vi "VIRefToJson.vi"(8 "error (in)":errorcluster, 10 "Destination Directory":path, 11 "vi reference":refnum<vi>) -> (0 "error out":errorcluster, 2 "JSON File Path":path, 3 "JSON":string)   [LabVIEW 2017]
panel:
  out "resulting string":string
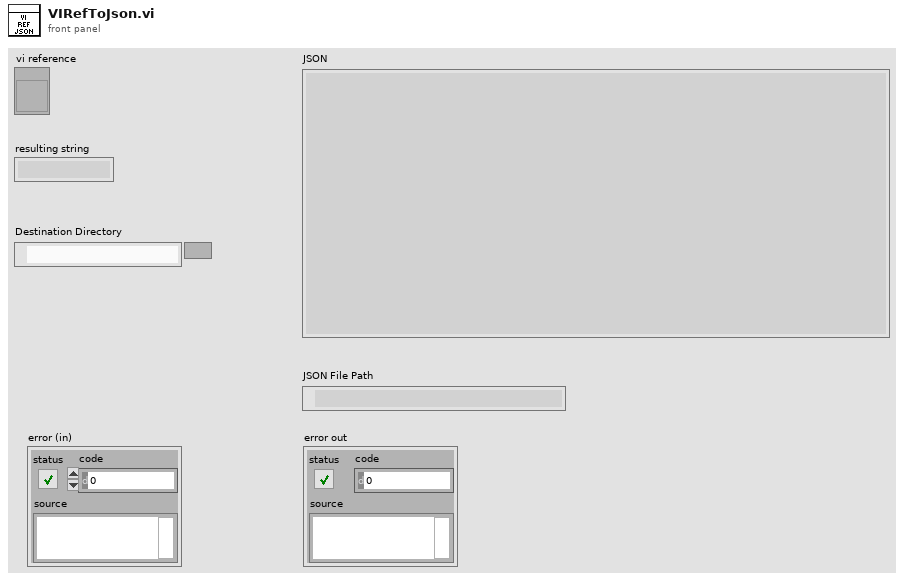
[diagram p1: front panel]
types:
  T1 = enum32{"invalid VI type", "Standard VI", "Control VI", "Global VI", "Polymorphic VI", "Configuration VI", "SubSystem", "Facade VI", "Method VI", "Statechart Diagram VI"}
  T2 = cluster{"VIPath":path, "Menu Name":string, "Selector Name":string}[]
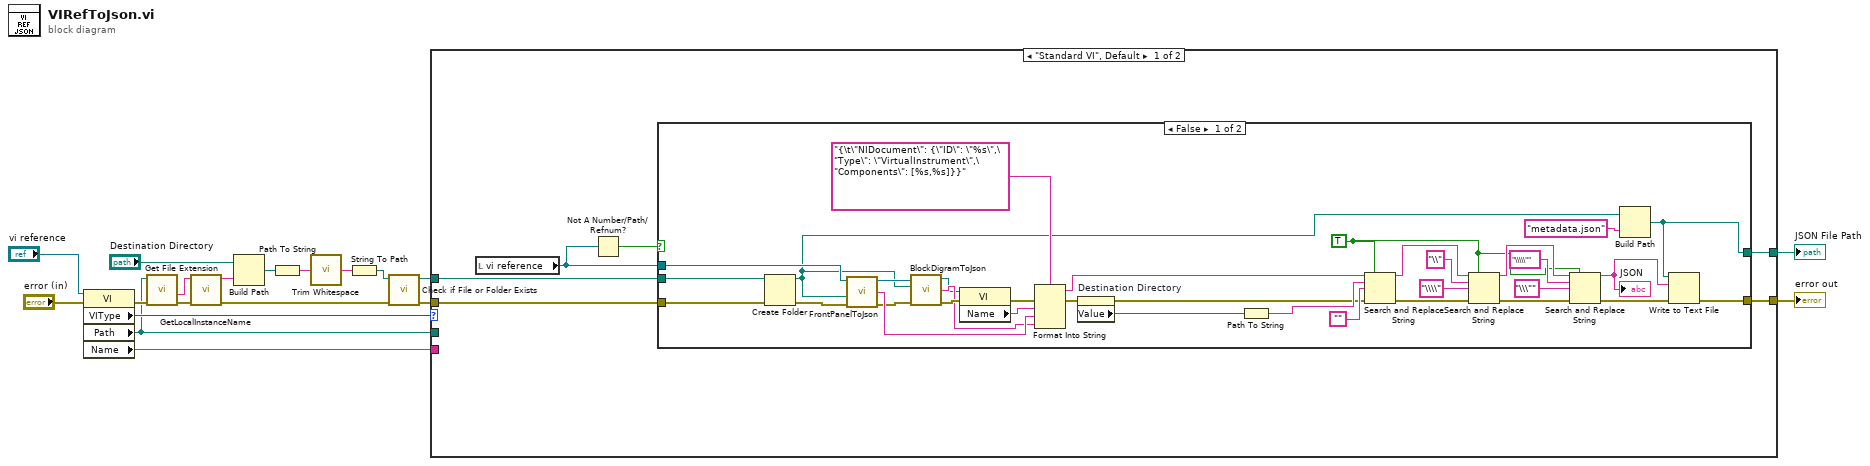
[diagram p0: block diagram]
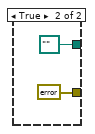
[diagram p2: hidden frame]
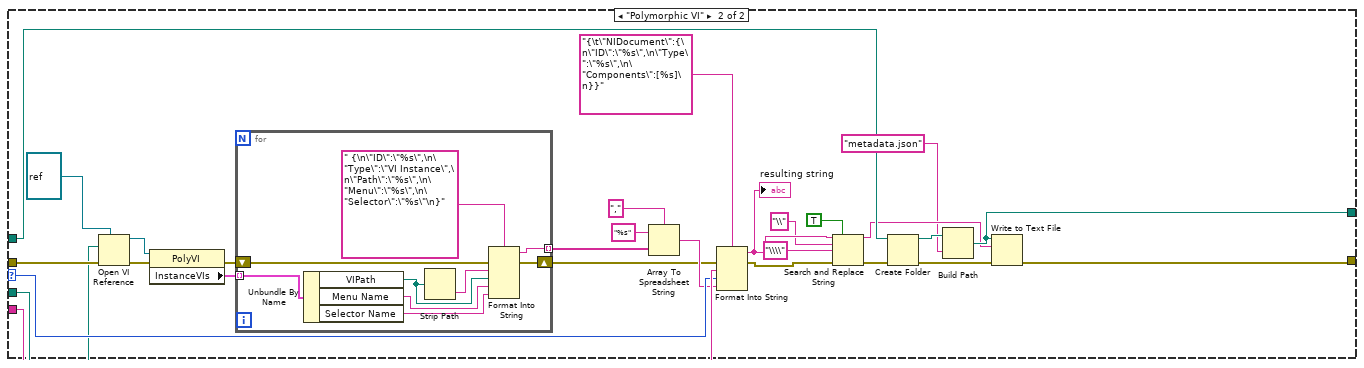
[diagram p3: hidden frame]
diagram:
  n1 = property class="VI"(reference="vi reference", error in="error (in)") -> (error out=w3:errorcluster, "VIType"=w7:T1, "Path"=w1:path, "Name"=w6:string)  [unwired: 1 out]
  n2 = call <vilib>:"Get File Extension.vi"("error in (no error)"=w3, "file"=w1) -> ("error out"=w17:errorcluster, "filename without extension"=w16:string)  [unwired: 5 in, 3 out]
  n3 = call "GetLocalInstanceName.vi"("error in (no error)"=w17, "result string in"=w16) -> ("error out"=w15:errorcluster, "result string out"=w12:string)  [unwired: 8 in]
  n4 = Build Path(base path="Destination Directory", name or relative path=w12) -> (appended path=w11:path)
  n5 = Path To String(path=w11) -> (string=w9:string)
  n6 = call <vilib>:"Trim Whitespace.vi"("string"=w9) -> ("trimmed string"=w10:string)  [unwired: 1 in]
  n7 = String To Path(string=w10) -> (path=w8:path)
  n8 = call <vilib>:"Check if File or Folder Exists.vi"("error in (no error)"=w15, "path"=w8) -> ("error out"=w2:errorcluster, "dup path"=w13:path)  [unwired: 7 in, 1 out]
  n9 = case shown="\"Standard VI\", Default" w7 {
    selector: w7 -> [_ w86]
    tunnel: [w25 w84] -> w19
    tunnel: [w24 w85] -> w18
    tunnel: w2 -> [w23 w88]
    tunnel: w13 -> [w22 w81]
    tunnel: w1 -> [_ w83]
    tunnel: w6 -> [_ w87]
    frame "Standard VI", Default {
      n10 = local read "vi reference"() -> (w20:refnum<vi>)
      n11 = Not A Number/Path/Refnum?(number/path/refnum=w20) -> (NaN/Path/Refnum?=w21:bool)
      n12 = case shown="False" w21 {
        tunnel: [w27 path ""] -> w25
        tunnel: [w59 errorcluster {"status"=FALSE, "code"=0, "source"=""} ("error out")] -> w24
        tunnel: w23 -> [w58 _]
        tunnel: w22 -> [w26 _]
        tunnel: w20 -> [w57 _]
        frame False {
          w34 = TRUE ("replace all? (F)")
          n13 = Create Folder(path (use dialog)=w26, error in=w58) -> (created path=w29:path, error out=w45:errorcluster)  [unwired: 1 in, 1 out]
          n14 = call "FrontPanelToJson.vi"("error in"=w45, "VI Path"=w29, "VI in"=w57) -> ("error out"=w44:errorcluster, "VI out"=w42:refnum<vi>, "JSON"=w46:string)  [unwired: 5 in]
          n15 = call "BlockDigramToJson.vi"("error in"=w44, "created path"=w29, "VI in"=w42) -> ("error out"=w43:errorcluster, "VI out"=w40:refnum<vi>, "JSON"=w41:string)  [unwired: 5 in]
          n16 = property class="VI"(reference=w40, error in=w43) -> (error out=w51:errorcluster, "Name"=w47:string)  [unwired: 1 out]
          n17 = Format Into String(format string="{\t\"NIDocument\": {\"ID\": \"%s\",\"Type\": \"VirtualInstrument\",\"Components\": [%s,%s]}}", error in=w51, w47, w46, w41) -> (resulting string=w53:string, error out=w31:errorcluster)  [unwired: 1 in]
          n18 = property on="Destination Directory" class="Path"(error in=w31) -> (error out=w30:errorcluster, "Value"=w32:path)  [unwired: 1 in, 1 out]
          n19 = Path To String(path=w32) -> (string=w48:string)
          n20 = Search and Replace String(replace all?=w34, input string=w53, search string=w48, replace string="", error in=w30) -> (result string=w54:string, error out=w50:errorcluster)  [unwired: 3 in, 2 out]
          n21 = Search and Replace String(replace all?=w34, input string=w54, search string="\\", replace string="\\\\" ("replace string (\"\")"), error in=w50) -> (result string=w39:string, error out=w35:errorcluster)  [unwired: 3 in, 2 out]
          n22 = Search and Replace String(replace all?=w34, input string=w39, search string="\\\\\"", replace string="\\\"" ("replace string (\"\")"), error in=w35) -> (result string=w38:string, error out=w33:errorcluster)  [unwired: 3 in, 2 out]
          "JSON" <- w38
          n23 = Build Path(base path=w29, name or relative path="metadata.json" ("string")) -> (appended path=w27:path)
          n24 = Write to Text File(file (use dialog)=w27, text=w38, error in=w33) -> (error out=w59:errorcluster)  [unwired: 1 in, 2 out]
        }
        frame True {
        }
      }
    }
    frame "Polymorphic VI" {
      n25 = Open VI Reference(type specifier VI Refnum (for type only)=refnum<vi> refnum, vi path=w83, error in (no error)=w88) -> (vi reference=w82:refnum<vi>, error out=w80:errorcluster)  [unwired: 3 in]
      n26 = property class="PolyVI"(reference=w82, error in=w80) -> (error out=w73:errorcluster, "InstanceVIs"=w79:T2)  [unwired: 1 out]
      n27 = for {
        tunnel: w79 -> [w98] mode=indexing
        tunnel: [w94] -> w78 mode=indexing
        shift-right: [w91] -> w74
        shift-left: w73 -> [w90]
        n28 = Unbundle By Name(w98) -> ("VIPath"=w93:path, "Menu Name"=w96:string, "Selector Name"=w95:string)
        n29 = Strip Path(path=w93) -> (name=w92:string)  [unwired: 1 out]
        n30 = Format Into String(format string=" {\n\"ID\":\"%s\",\n\"Type\":\"VI Instance\",\n\"Path\":\"%s\",\n\"Menu\":\"%s\",\n\"Selector\":\"%s\"\n}", error in=w90, w92, w93, w96, w95) -> (resulting string=w94:string, error out=w91:errorcluster)  [unwired: 1 in]
      }
      n31 = Array To Spreadsheet String(delimiter (Tab)=",", array=w78, 3:"%s" ("format string")) -> (spreadsheet string=w75:string)
      n32 = Format Into String(format string="{\t\"NIDocument\":{\n\"ID\":\"%s\",\n\"Type\":\"%s\",\n\"Components\":[%s]\n}}", error in=w74, w87, w86, w75) -> (resulting string=w71:string, error out=w65:errorcluster)  [unwired: 1 in]
      "resulting string" <- w71
      n33 = Search and Replace String(replace all?=TRUE ("replace all? (F)"), input string=w71, search string="\\", replace string="\\\\" ("replace string (\"\")"), error in=w65) -> (result string=w68:string, error out=w64:errorcluster)  [unwired: 3 in, 2 out]
      n34 = Create Folder(path (use dialog)=w81, error in=w64) -> (created path=w66:path, error out=w62:errorcluster)  [unwired: 1 in, 1 out]
      n35 = Build Path(base path=w66, name or relative path="metadata.json" ("string")) -> (appended path=w84:path)
      n36 = Write to Text File(file (use dialog)=w84, text=w68, error in=w62) -> (error out=w85:errorcluster)  [unwired: 1 in, 2 out]
    }
  }
  "JSON File Path" <- w19
  "error out" <- w18
